vi "radio_reception_mode.vi"(8 "error in":errorcluster, 11 "VISA in":refnum<visa-resource-name>) -> (0 "error out":errorcluster, 1 "error":bool, 3 "VISA out":refnum<visa-resource-name>)   [LabVIEW 2011]
panel:
  out "read buffer":string
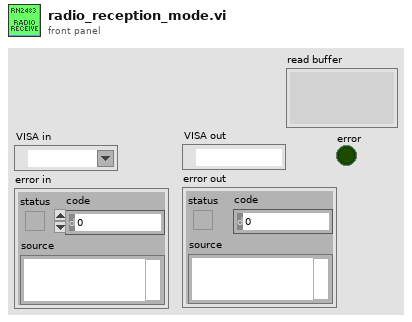
[diagram p1: front panel]
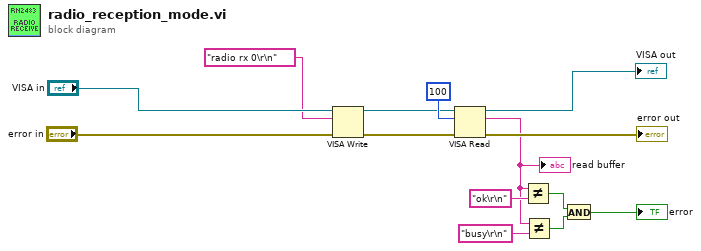
[diagram p0: block diagram]
diagram:
  n1 = VISA Write(VISA resource name="VISA in", write buffer="radio rx 0\r\n" ("string to write"), error in (no error)="error in") -> (VISA resource name out=w9:refnum<visa-resource-name>, error out=w8:errorcluster)  [unwired: 1 out]
  n2 = VISA Read(VISA resource name=w9, byte count=u32 100, error in (no error)=w8) -> (VISA resource name out=→"VISA out":refnum<visa-resource-name>, read buffer=w5:string, error out=→"error out":errorcluster)  [unwired: 1 out]
  "read buffer" <- w5
  n3 = Not Equal?(x=w5, y="ok\r\n") -> (x != y?=w3:bool)
  n4 = Not Equal?(x=w5, y="busy\r\n") -> (x != y?=w2:bool)
  n5 = And(x=w3, y=w2) -> (x .and. y?=→"error":bool)
